vi "polarToCartesian.vi"(2 "Angle (deg)":dbl, 3 "Magnitude (r)":dbl) -> (0 "y":dbl, 1 "x":dbl)   [LabVIEW 2016]
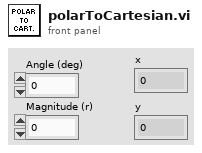
[diagram p1: front panel]
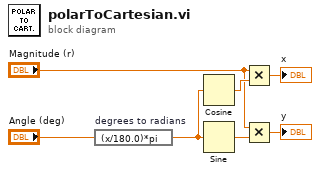
[diagram p0: block diagram]
diagram:
  n1 = expression code="(x/180.0)*pi" "degrees to radians"("Angle (deg)") -> (w1:dbl)
  n2 = Cosine(x=w1) -> (cos(x)=w5:dbl)
  n3 = Sine(x=w1) -> (sin(x)=w4:dbl)
  n4 = Multiply(x="Magnitude (r)", y=w5) -> (x*y=→"x":dbl)
  n5 = Multiply(x="Magnitude (r)", y=w4) -> (x*y=→"y":dbl)
